vi "initiateTSR.vi"(0 "reference in":refnum<class "excelFile.lvclass">, 5 "error in (no error)":errorcluster) -> (14 "reference out":refnum<class "excelFile.lvclass">, 19 "error out":errorcluster)   [LabVIEW 2016, in "excelFile.lvclass"]
doc: "Initiate the ranges where the data must be populated into the TSR excel files."
uses:
  excelFile.lvclass
  SYS/File Controller_llb/File Controller.lvclass
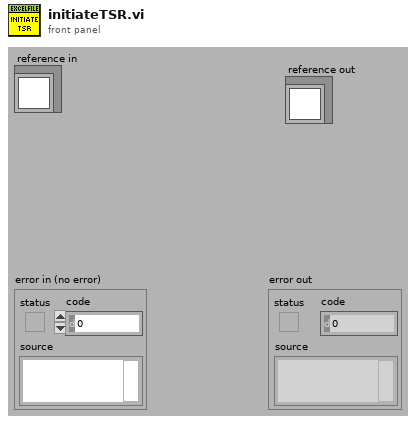
[diagram p1: front panel]
types:
  T1 = cluster{"number":i32[], "date":i32[], "company":i32[], "department":i32[], "address":i32[], "city":i32[], "post_code":i32[], "country":i32[], "contact":i32[], "product":i32[], "serial_number":i32[], "start_time":i32[], "end_time":i32[], "pmc_number":i32[], "issue_description":i32[], "actions":i32[], "defective_parts":i32[], "spare+parts":i32[], "labour_hours":i32[], "labour_price":i32[], "shipping":i32[], "discount":i32[]}
  T2 = typedef "excelFile.lvclass/ObjectAttributesRef.ctl" = refnum<data-value>
  T3 = cluster{"number":string, "TSR_path":path, "service_path":path, "email_to":string}
  T4 = typedef "excelFile.lvclass/ObjectAttributes.ctl" = cluster{"MyAttribute":dbl, "path":string, "Refnum Excel":cluster{"Excel._Application":refnum<k7>, "Workbooks":refnum<k7>, "Open":refnum<k7>}, "data":string[][][], "save":bool, "fileType":T5, "rowsColor":u32[], "python_ref":refnum<class "python.lvclass">, "items_rows":i32[], "excel_range":i32[][], "TSR":cluster{"number":string, "TSR_path":path, "service_path":path, "email_to":string}, "excel_already_opened?":bool, "file_already_opened?":bool, "excel_protected_opened?":bool, "Refnum Cluster Worksheets":cluster{"Excel._Application":refnum<k7>, "Workbooks":refnum<k7>, "Open":refnum<k7>, "Worksheets":refnum<k7>, "Excel._Worksheet":refnum<k7>}, "#_rows_defective":i32, "#_rows_spare":i32}
  T5 = typedef "excelFile.lvclass/fileType.ctl" = enum16{"devices", "items", "partsTracking", "TSR"}
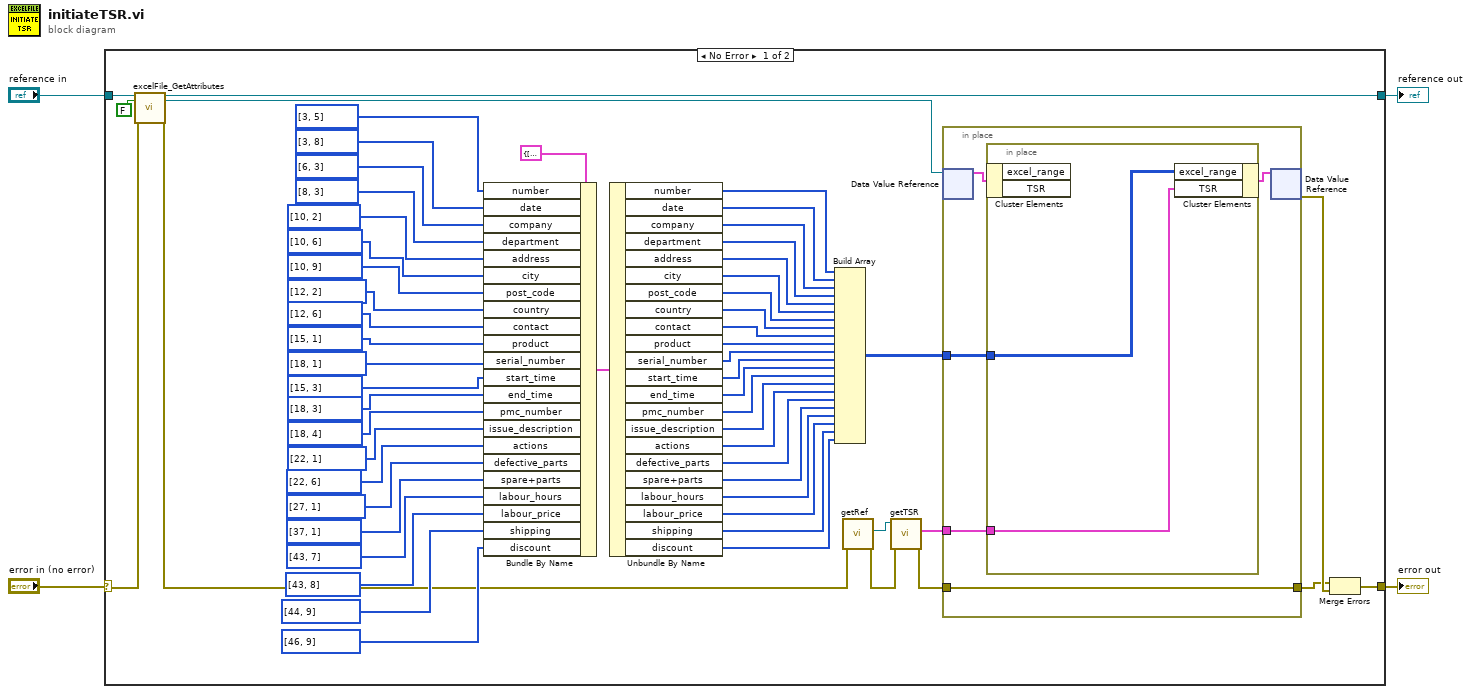
[diagram p0: block diagram]
diagram:
  n1 = case shown="No Error" "error in (no error)" {
    selector: "error in (no error)" -> [w59 w73]
    tunnel: [w64 w73] -> w3
    tunnel: [w58 w72] -> w1
    tunnel: "reference in" -> [w61 w72]
    frame No Error {
      n2 = call "excelFile_GetAttributes.vi"("reference in"=w61, "return data? (T)"=FALSE, "error in (no error)"=w59) -> ("reference out"=w58:refnum<class "excelFile.lvclass">, "attributes ref"=w57:T2, "error out"=w11:errorcluster)  [unwired: 13 in, 1 out]
      n3 = Bundle By Name(cluster=T1 {"number"=[], "date"=[], "company"=[], "department"=[], "address"=[], "city"=[], "post_code"=[], "country"=[], "contact"=[], "product"=[], "serial_number"=[], "start_time"=[], "end_time"=[], "pmc_number"=[], "issue_description"=[], "actions"=[], "defective_parts"=[], "spare+parts"=[], "labour_hours"=[], "labour_price"=[], "shipping"=[], "discount"=[]} ("excel_range"), "number"=i32[] [3, 5], "date"=i32[] [3, 8] ("number"), "company"=i32[] [6, 3] ("number"), "department"=i32[] [8, 3] ("number"), "address"=i32[] [10, 2] ("number"), "city"=i32[] [10, 6] ("number"), "post_code"=i32[] [10, 9] ("number"), "country"=i32[] [12, 2] ("number"), "contact"=i32[] [12, 6] ("number"), "product"=i32[] [15, 1] ("number"), "serial_number"=i32[] [18, 1] ("number"), "start_time"=i32[] [15, 3] ("number"), "end_time"=i32[] [18, 3] ("number"), "pmc_number"=i32[] [18, 4] ("number"), "issue_description"=i32[] [22, 1] ("number"), "actions"=i32[] [22, 6] ("number"), "defective_parts"=i32[] [27, 1] ("number"), "spare+parts"=i32[] [37, 1] ("number"), "labour_hours"=i32[] [43, 7] ("number"), "labour_price"=i32[] [43, 8] ("number"), "shipping"=i32[] [44, 9] ("number"), "discount"=i32[] [46, 9] ("number")) -> (w35:T1)
      n4 = Unbundle By Name(w35) -> ("number"=w34:i32[], "date"=w33:i32[], "company"=w32:i32[], "department"=w31:i32[], "address"=w30:i32[], "city"=w29:i32[], "post_code"=w28:i32[], "country"=w27:i32[], "contact"=w26:i32[], "product"=w25:i32[], "serial_number"=w24:i32[], "start_time"=w23:i32[], "end_time"=w22:i32[], "pmc_number"=w21:i32[], "issue_description"=w20:i32[], "actions"=w19:i32[], "defective_parts"=w18:i32[], "spare+parts"=w17:i32[], "labour_hours"=w16:i32[], "labour_price"=w15:i32[], "shipping"=w14:i32[], "discount"=w5:i32[])
      n5 = Build Array(w34, w33, w32, w31, w30, w29, w28, w27, w26, w25, w24, w23, w22, w21, w20, w19, w18, w17, w16, w15, w14, w5) -> (w13:i32[][])
      n6 = call "getRef.vi"("error in (no error)"=w11) -> ("error out"=w10:errorcluster, "File Controller_ref"=w12:refnum<class "File Controller.lvclass">)  [unwired: 9 in]
      n7 = call "getTSR.vi"("error in (no error)"=w10, "reference in"=w12) -> ("error out"=w9:errorcluster, "TSR"=w8:T3)  [unwired: 7 in, 1 out]
      n8 = in-place {
        in-place-border: w9 -> [w67]
        in-place-border: [w67] -> w62
        in-place-border: w13 -> [w66]
        in-place-border: w8 -> [w65]
        n9 = in-place-dvr #1(w57) -> (w68:T4)  [unwired: 1 out]
        n10 = in-place {
          in-place-border: w66 -> [w71]
          in-place-border: w65 -> [w70]
          n11 = in-place-cluster #2(w68) -> ()  [unwired: 2 out]
          n12 = in-place-cluster #2("excel_range"=w71, "TSR"=w70) -> (w69:T4)
        }
        n13 = in-place-dvr #1(w69) -> (w63:errorcluster)  [unwired: 1 out]
      }
      n14 = Merge Errors(w62, w63) -> (w64:errorcluster)
    }
    frame Error {
    }
  }
  "error out" <- w3
  "reference out" <- w1
